vi "Init.vi"(5 "Difficulty":dbl, 6 "Self Index in":i32, 7 "Players number in":i32, 9 "Right width goal in":u32, 10 "Bounds in":T1) -> (0 "error out":errorcluster, 3 "AI Manager out":refnum<class "AI Manager.lvclass">)   [LabVIEW 2024, in "AI Manager.lvclass"]
doc: "MIT Licence\nCopyright (c) 2024 David Grollier"
uses:
  AI Manager.lvclass
  <vilib>/Utility/miscctls.llb/LVBoundsTypeDef.ctl
  AI Manager.lvclass/AI Manager.ctl
  <vilib>/Utility/error.llb/Error Cluster From Error Code.vi
  <vilib>/ErrorRing/Error Ring.xnode
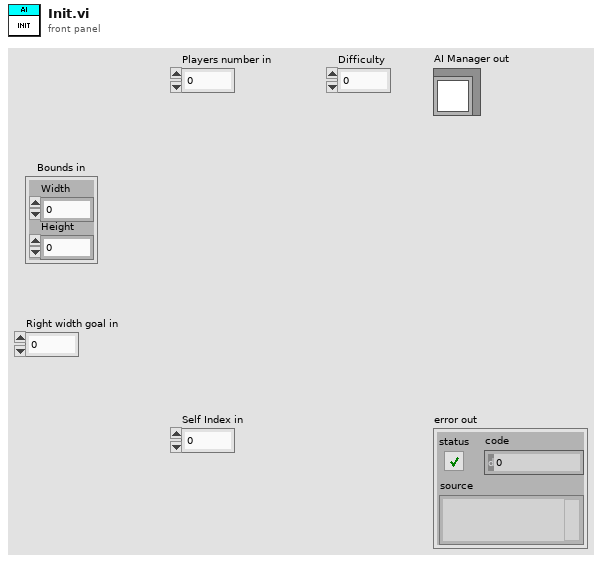
[diagram p1: front panel]
types:
  T1 = typedef "LVBoundsTypeDef.ctl" = cluster{"Width":u32, "Height":u32}
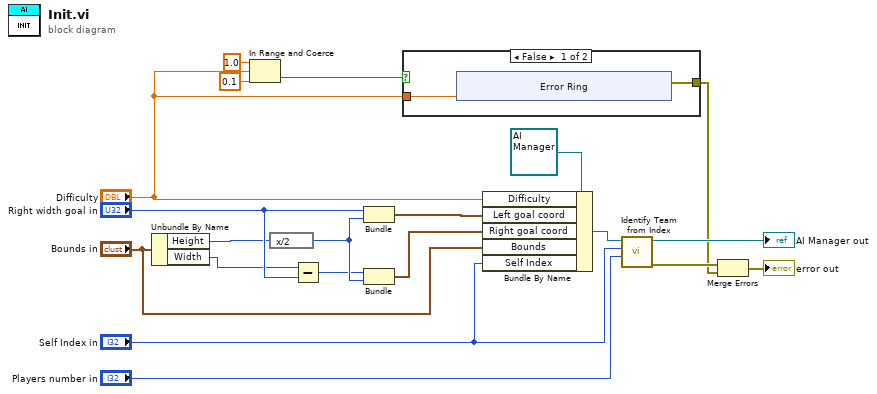
[diagram p0: block diagram]
diagram:
  n1 = Unbundle By Name("Bounds in") -> ("Height"=w14:u32, "Width"=w13:u32)
  n2 = In Range and Coerce(upper limit=1.0, x="Difficulty", lower limit=0.1) -> (In Range?=w5:bool)  [unwired: 1 out]
  n3 = expression code="x/2"(w14) -> (w17:u32)
  n4 = Subtract(x=w13, y="Right width goal in") -> (x-y=w15:u32)
  n5 = Bundle("Right width goal in"="Right width goal in", "Height"=w17) -> (w19:cluster{"Right width goal in":u32, "Height":u32})  [unwired: 1 in]
  n6 = Bundle(w15, "Height"=w17) -> (w18:cluster{u32, "Height":u32})  [unwired: 1 in]
  n7 = case shown="False" w5 {
    tunnel: [w22 _] -> w3
    tunnel: "Difficulty" -> [w21 _]
    frame False {
      n8 = xnode "Error Ring"("parameter 0"=w21) -> ("error out"=w22:errorcluster)
    }
    frame True {
    }
  }
  n9 = Bundle By Name(cluster=refnum<class "AI Manager.lvclass"> refnum ("AI Manager in"), "Difficulty"="Difficulty", "Left goal coord"=w19, "Right goal coord"=w18, "Bounds"="Bounds in", "Self Index"="Self Index in") -> (w11:refnum<class "AI Manager.lvclass">)
  n10 = call "Identify Team from Index.vi"("Players number in"="Players number in", "Self index in"="Self Index in", "AI Manager in"=w11) -> ("error out"=w4:errorcluster, "AI Manager out"=→"AI Manager out":refnum<class "AI Manager.lvclass">)  [unwired: 7 in]
  n11 = Merge Errors(w4, w3) -> (→"error out":errorcluster)
